vi "MISC Wait with Data Flow.vi"(6 "Wait Mode (Timer)":T1, 7 "Notifier":refnum<notifier>, 8 "Error In (no error)":errorcluster, 10 "Ignore Previous (F)":bool, 11 "Wait Time (500ms)":u32=500) -> (0 "Error Out":errorcluster, 1 "Aborted":bool, 3 "Timer Value (ms)":u32)   [LabVIEW 2017]
uses:
  Type Defs/MISC MS Timer Wait Mode Enum.ctl
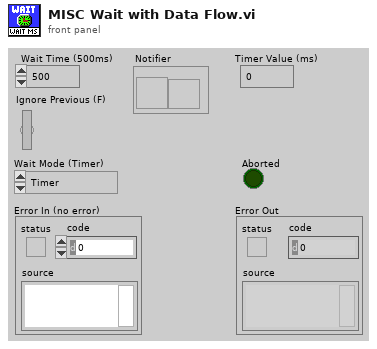
[diagram p1: front panel]
types:
  T1 = typedef "MISC MS Timer Wait Mode Enum.ctl" = enum16{"Timer", "Notifier"}
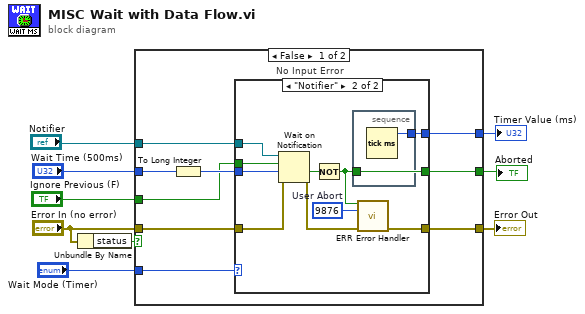
[diagram p0: block diagram]
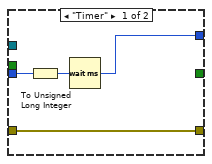
[diagram p2: hidden frame]
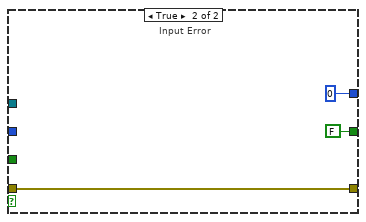
[diagram p3: hidden frame]
diagram:
  n1 = Unbundle By Name("Error In (no error)") -> ("status"=w9:bool)
  n2 = case shown="False" w9 {
    tunnel: "Wait Time (500ms)" -> [w11 _]
    tunnel: [w17 w36] -> w7
    tunnel: "Error In (no error)" -> [w18 w36]
    tunnel: "Notifier" -> [w16 _]
    tunnel: [w10 FALSE] -> w5
    tunnel: [w15 u32 0 ("millisecond timer value")] -> w4
    tunnel: "Ignore Previous (F)" -> [w13 _]
    tunnel: "Wait Mode (Timer)" -> [w12 _]
    frame False {
      # "No Input Error"
      n3 = To Long Integer(number=w11) -> (32bit integer=w14:i32)
      n4 = case shown="\"Notifier\"" w12 {
        tunnel: w14 -> [w20 w29]
        tunnel: w16 -> [_ w32]
        tunnel: w18 -> [w22 w31]
        tunnel: [w22 w23] -> w17
        tunnel: [_ w25] -> w10
        tunnel: w13 -> [_ w30]
        tunnel: [w21 w28] -> w15
        frame "Timer" {
          n5 = To Unsigned Long Integer(number=w20) -> (unsigned 32bit integer=w19:u32)
          n6 = Wait (ms)(milliseconds to wait=w19) -> (millisecond timer value=w21:u32)
        }
        frame "Notifier" {
          w24 = 9876  # User Abort
          n7 = Wait on Notification(notifier=w32, ignore previous (F)=w30, timeout in ms (-1)=w29, error in (no error)=w31) -> (timed out?=w26:bool, error out=w27:errorcluster)  [unwired: 2 out]
          n8 = Not(x=w26) -> (.not. x?=w25:bool)
          n9 = stacked-sequence {
            tunnel: [w33] -> w28
            tunnel: w25 -> [_]
            frame #0 {
              n10 = Tick Count (ms)() -> (millisecond timer value=w33:u32)
            }
          }
          n11 = call "ERR Error Handler.vi"("Error Status"=w25, "Error Code"=w24, "Error In (no error)"=w27) -> ("Error Out"=w23:errorcluster)  [unwired: 3 in, 9 out]
        }
      }
    }
    frame True {
      # "Input Error"
    }
  }
  "Error Out" <- w7
  "Aborted" <- w5
  "Timer Value (ms)" <- w4
